vi "Update Root Message.vi"(8 "error in (no error)":errorcluster, 10 "Message":string, 11 "Nested in":refnum<class "Nested.lvclass">) -> (0 "error out":errorcluster, 3 "Nested out":refnum<class "Nested.lvclass">)   [LabVIEW 2025, in "Nested.lvlib" / "Nested.lvclass"]
uses:
  Nested.lvclass
  C:/Program Files/National Instruments/LabVIEW 2025/vi.lib/ActorFramework/Actor/Actor.lvclass
  <vilib>/ActorFramework/Actor/Actor.lvclass/Actor.ctl
  Root Interface/Root Interface Messages/Update Root Message Msg/Update Root Message Msg.lvclass/Update Root Message Msg.ctl
  <vilib>/ActorFramework/Message Enqueuer/Message Enqueuer.lvclass/Message Enqueuer.ctl
  <vilib>/ActorFramework/Message Enqueuer/Enqueue.vi
  Root Interface/Root Interface Messages/Update Root Message Msg/Update Root Message Msg.lvclass
  C:/Program Files/National Instruments/LabVIEW 2025/vi.lib/ActorFramework/Message/Message.lvclass
  <vilib>/ActorFramework/Message Priority Queue/Priority Enqueue.vi
  Nested.lvclass/Nested.ctl
  <vilib>/ActorFramework/Actor/Actor.lvclass
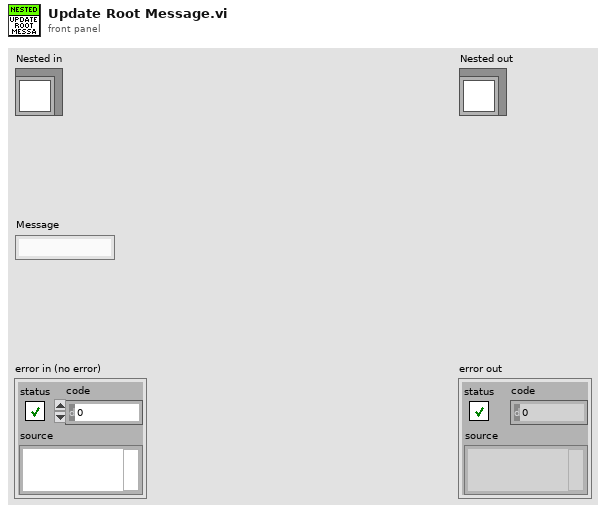
[diagram p1: front panel]
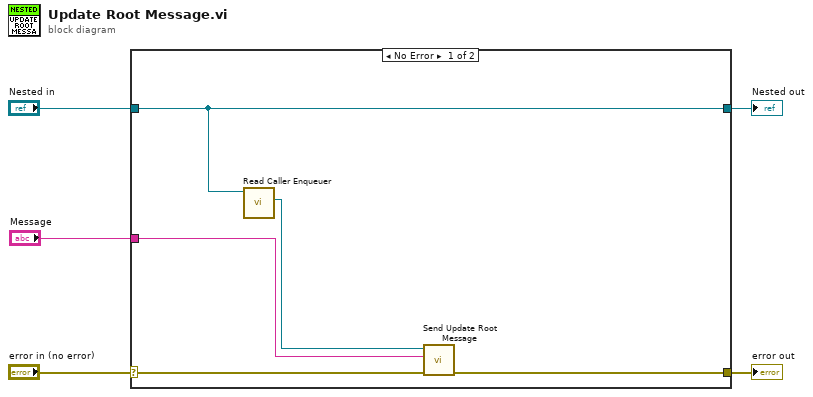
[diagram p0: block diagram]
diagram:
  n1 = case shown="No Error" "error in (no error)" {
    selector: "error in (no error)" -> [w8 w12]
    tunnel: [w9 w12] -> w4
    tunnel: [w10 w11] -> w2
    tunnel: "Nested in" -> [w10 w11]
    tunnel: "Message" -> [w6 _]
    frame No Error {
      n2 = call <vilib>:"Read Caller Enqueuer.vi"("Actor"=w10) -> ("Caller Enqueuer"=w7:refnum<class "Message Enqueuer.lvclass">)  [unwired: 10 in]
      n3 = call "Send Update Root Message.vi"("error in (no error)"=w8, "Message"=w6, "Message Enqueuer"=w7) -> ("error out"=w9:errorcluster)  [unwired: 7 in, 1 out]
    }
    frame Error {
    }
  }
  "error out" <- w4
  "Nested out" <- w2
